vi "HEX字符串转十六进制数组.vi"(11 "字符":string) -> (3 "数组":u8[](array[numeric]))   [LabVIEW 2015]
panel:
  out "长度":i32
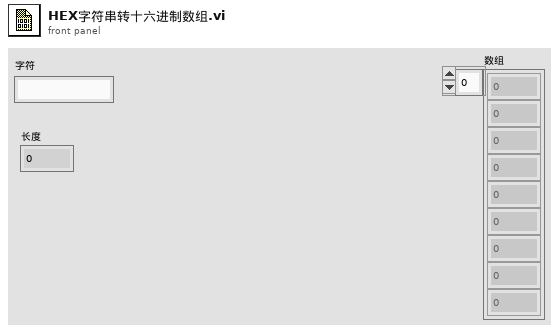
[diagram p1: front panel]
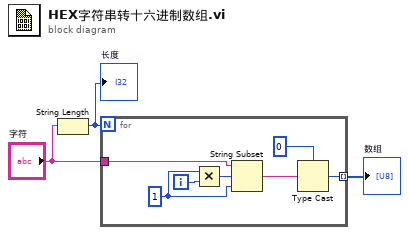
[diagram p0: block diagram]
diagram:
  n1 = String Length(string="字符") -> (length=w2:i32)
  "长度" <- w2
  n2 = for {
    N: w2 -> [_]
    tunnel: "字符" -> [w7]
    tunnel: [w4] -> w3 mode=indexing
    i -> [w10]
    w9 = 1 ("长度（剩余）")
    n3 = Multiply(x=w9, y=w10) -> (x*y=w8:i32)
    n4 = String Subset(string=w7, offset (0)=w8, length (rest)=w9) -> (substring=w6:string)
    n5 = Type Cast(type=u8 0, x=w6) -> (*(type *) &x=w4:u8)
  }
  "数组" <- w3
